vi "Periodic Tasks.vi"(8 "error in (no error)":errorcluster) -> ()   [LabVIEW 2019]
doc: "This VI runs in parallel to other tasks. It can contain as many user-defined periodic loops as you need. These can carry out PID or other sorts of timed response."
uses:
  <vilib>/Rock Robotics/WPI/ThirdParty/Phoenix-LabVIEW/Motor Controller/Controls/CTRE_Phoenix_MotorControl_ControlMode.ctl
  <vilib>/Rock Robotics/WPI/Solenoid/WPI_SolenoidValue.ctl
  <vilib>/Rock Robotics/WPI/ThirdParty/Sensors/navX/_TypeDefs/FRIC_navX_DeviceNumbersTypeDef.ctl
  <vilib>/Rock Robotics/WPI/ThirdParty/Phoenix-LabVIEW/Motor Controller/Controls/CTRE_Phoenix_MotorControl_FeedbackDevice.ctl
  <vilib>/Rock Robotics/WPI/DriverStation/WPI_DriverStationRobotMode2.ctl
  Corsair_V1/Team Code/Climber Routine.ctl
  Corsair_V1/Team Code/Ball Routine.ctl
  TurretMode.ctl
  LabVIEW_is_Under_Control.lib/Util/Toggle/Change Detect.vi
  LabVIEW_is_Under_Control.lib/Util/Toggle/Change Detect Boolean.vi
  <vilib>/Rock Robotics/WPI/Utilities/WPI_GetSetVariantRefNum.vi
  MotorsGlobal.vi
  JoysticksGlobal.vi
  <vilib>/Rock Robotics/Network Tables/NT Read Number.vi
  <vilib>/Rock Robotics/WPI/Solenoid/WPI_SolenoidSetEnum.vi
  <vilib>/Rock Robotics/WPI/ThirdParty/Phoenix-LabVIEW/Motor Controller/Get/CTRE_Phoenix_MotorController_GetSelectedSensorData.vi
  Robot Global Data.vi
  <vilib>/Rock Robotics/Network Tables/NT Write Number.vi
  <vilib>/Rock Robotics/WPI/ThirdParty/Phoenix-LabVIEW/Motor Controller/Get/CTRE_Phoenix_MotorController_GetVoltage.vi
  Ball counter.ctl
panel:
  in  "Distancia de longshot":dbl
  in  "Corsair Control":T1(tab)
  in  "EnableFWPID":bool
  out "Voltage":dbl
  out "Voltage Output":cluster{"Percent Output":dbl}(graph)
  out "Velocity PIDF":T2(graph)
  in  "I Zone":dbl
  in  "D":dbl
  in  "I":dbl
  in  "P":dbl=1.0
  in  "kF":dbl=0.031
  in  "FWSetpoint":dbl
  out "Flywheel Encoder":i32
  out "LTAGainsON?":bool
  in  "Inner Goal Height":dbl=2.49
  in  "Camera Angle":dbl=20.0
  out "Distancia do Goal":dbl
  in  "Camera Height":dbl=0.5599999999999999
  out "Turret PID":cluster{"Setpoint":dbl, "Process variable":dbl}(graph)
  in  "TAGains":T3={"proportional gain (Kc)"=0.4, "integral time (Ti, min)"=0.0, "derivative time (Td, min)"=0.0} {"derivative time (Td, min)" format="%.3f"; "integral time (Ti, min)" format="%.3f"; "proportional gain (Kc)" format="%.3f"}
  in  "HTARange":cluster{"output high":dbl, "output low":dbl}={"output high"=0.5, "output low"=-0.5} {"output low" format="%.2f"; "output high" format="%.2f"}
  in  "MaxAngle":dbl=1000.0
  in  "TASetpoint":dbl
  in  "Minimum command":dbl=0.05
  out "Turret Out":dbl
  in  "TADisable Range":dbl
  in  "TAIntegral Range":dbl=10000.0
  in  "LTARange":cluster{"output high":dbl, "output low":dbl}={"output high"=0.35, "output low"=-0.35} {"output low" format="%.2f"; "output high" format="%.2f"}
  in  "MTARange":cluster{"output high":dbl, "output low":dbl}={"output high"=0.19999999999999996, "output low"=-0.19999999999999996} {"output low" format="%.2f"; "output high" format="%.2f"}
  in  "LTAGains":T3={"proportional gain (Kc)"=0.4, "integral time (Ti, min)"=0.0, "derivative time (Td, min)"=0.0} {"derivative time (Td, min)" format="%.3f"; "integral time (Ti, min)" format="%.3f"; "proportional gain (Kc)" format="%.3f"}
  in  "Setpoint Climber":dbl=-110.0
  in  "Reset Encoders":bool
  out "Current 4":dbl
  out "Motor Temperature 4":u8
  out "Current 3":dbl
  out "Motor Temperature 3":u8
  out "Current 2":dbl
  out "Motor Temperature 2":u8
  out "Current":dbl
  out "Motor Temperature":u8
  out "Left Encoder":dbl
  out "Right Encoder":dbl
  in  "Sensitivty":dbl=1.5
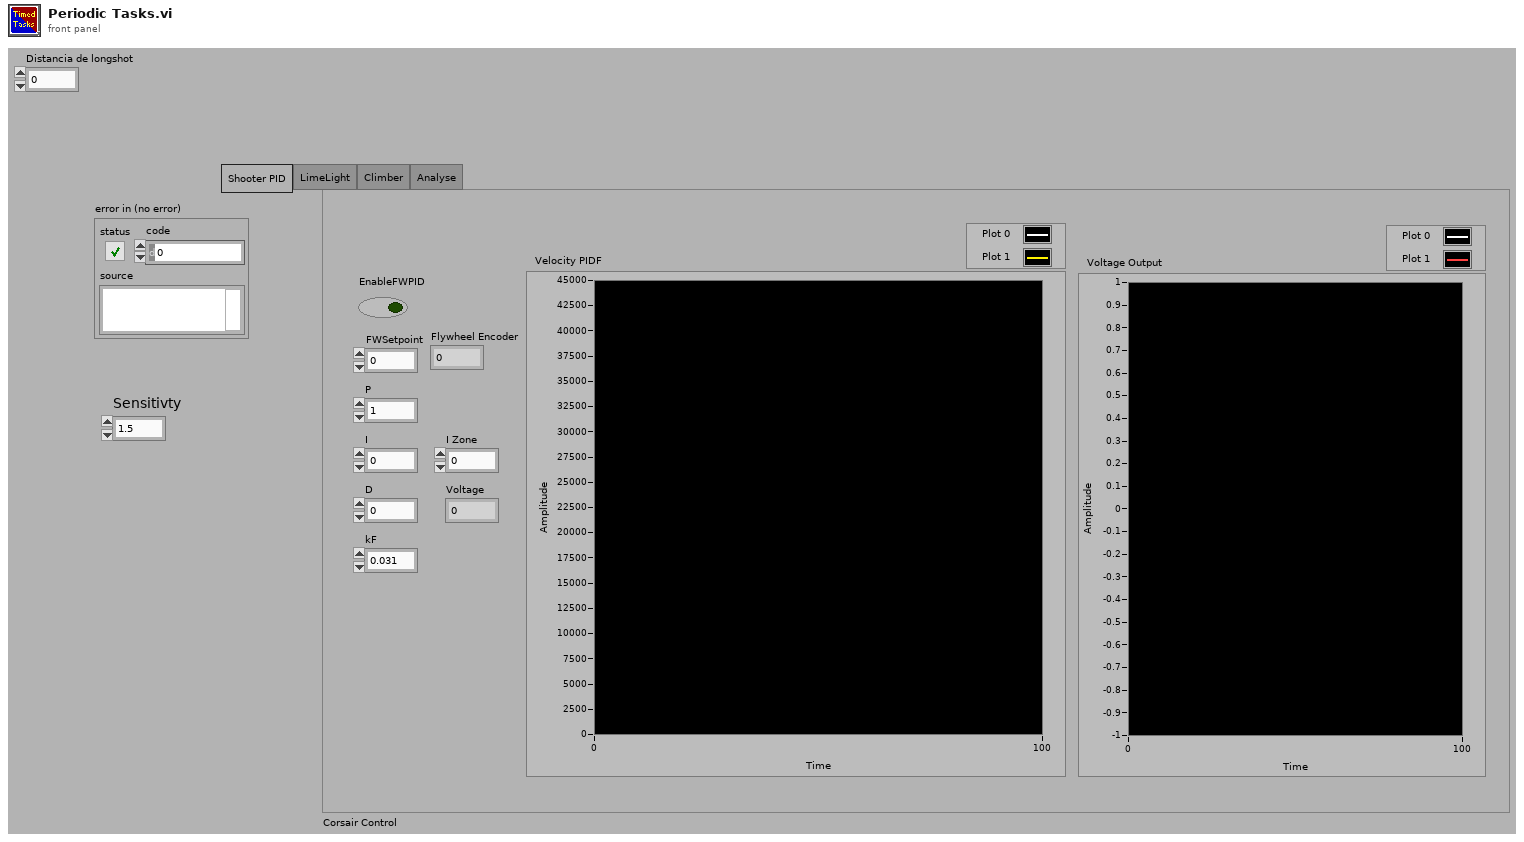
[diagram p1: front panel]
types:
  T1 = enum32{"Shooter PID", "LimeLight", "Climber", "Analyse"}
  T2 = cluster{"FWSetpoint":dbl, "Velocity (Raw Sensor Units per 100 ms)":i32}
  T3 = cluster{"proportional gain (Kc)":dbl, "integral time (Ti, min)":dbl, "derivative time (Td, min)":dbl}
  T4 = typedef "WPI_EncoderDevRef.ctl" = cluster{"DevStatus":errorcluster, "EncoderIndex":T5, "CounterIndex":T6, "DistancePerCount":dbl, "Decoding Type":T7}
  T5 = typedef "FPGA_EncoderIdx.ctl" = enum8{"Enc 0", "Enc 1", "Enc 2", "Enc 3", "Enc 4", "Enc 5", "Enc 6", "Enc 7", "Invalid"}
  T6 = typedef "FPGA_CounterCtrSystemIndex.ctl" = enum8{"Ctr 0", "Ctr 1", "Ctr 2", "Ctr 3", "Ctr 4", "Ctr 5", "Ctr 6", "Ctr 7", "Invalid"}
  T7 = typedef "WPI_EncoderType.ctl" = enum16{"1x", "2x", "4x"}
  T8 = typedef "WPI_JoystickDevRef.ctl" = cluster{"Device":T9}
  T9 = typedef "WPI_JoystickDeviceEnum.ctl" = enum16{"USB 0", "USB 1", "USB 2", "USB 3", "USB 4", "USB 5"}
  T10 = typedef "WPI_MotorControlDeviceRef.ctl" = cluster{"DeviceStatus":errorcluster, "Type":T11, "PWM":cluster{"PWM Channel":T12, "DeadBand":T13}, "CAN":cluster{"Device Number":u8, "SetOutput VI Ref":variant, "GetOutput VI Ref":variant, "Enable VI Ref":variant, "Disable VI Ref":variant, "Data":variant}, "Invert":bool, "DIO PWM":cluster{"PWM \"Enable\" Channel":T12, "DIOChannel":T14, "PWM Rate":dbl}}
  T11 = typedef "WPI_MotorControlType.ctl" = enum16{"PWM", "CAN", "DIO PWM"}
  T12 = typedef "FPGA_DIOPWMChannel.ctl" = enum8{"PWM 0", "PWM 1", "PWM 2", "PWM 3", "PWM 4", "PWM 5", "PWM 6", "PWM 7", "PWM 8", "PWM 9", "PWM MXP 0", "PWM MXP 1", "PWM MXP 2", "PWM MXP 3", "PWM MXP 4", "PWM MXP 5", "PWM MXP 6", "PWM MXP 7", "PWM MXP 8", "PWM MXP 9", "Invalid"}
  T13 = typedef "WPI_PWMDeadband.ctl" = cluster{"Name":string, "maxPositivePwm":i32, "minPositivePwm":i32, "centerPwm":i32, "maxNegativePwm":i32, "minNegativePwm":i32, "angularRange":u16}
  T14 = typedef "FPGA_DIOChannel.ctl" = enum8{"DIO 0", "DIO 1", "DIO 2", "DIO 3", "DIO 4", "DIO 5", "DIO 6", "DIO 7", "DIO 8", "DIO 9", "DIO MXP 0", "DIO MXP 1", "DIO MXP 2", "DIO MXP 3", "DIO MXP 4", "DIO MXP 5", "DIO MXP 6", "DIO MXP 7", "DIO MXP 8", "DIO MXP 9", "DIO MXP 10", "DIO MXP 11", "DIO MXP 12", "DIO MXP 13", "DIO MXP 14", "DIO MXP 15", "SPI Port CS1", "SPI Port CS2", "SPI Port CS3", "SPI Port MISO", "SPI Port MOSI", "Invalid"}
  T15 = typedef "WPI_SolenoidDevRef.ctl" = cluster{"DevStatus":errorcluster, "Pneumatics Control Module":u8, "Forward Solenoid Channel":T16, "Reverse Solenoid Channel":T16}
  T16 = typedef "WPI_SolenoidChannel.ctl" = enum8{"Solenoid 0", "Solenoid 1", "Solenoid 2", "Solenoid 3", "Solenoid 4", "Solenoid 5", "Solenoid 6", "Solenoid 7", "Invalid"}
  T17 = typedef "WPI_SwitchDevRef.ctl" = cluster{"DevStatus":errorcluster, "DIO Channel":T14, "CntIndex":T6, "Normally Closed":bool}
  T18 = typedef "FRIC_navX_DeviceNumbersTypeDef.ctl" = enum16{"Dev0", "Dev1", "Dev2", "Dev3"}
  T19 = typedef "WPI_SolenoidValue.ctl" = enum16{"Off", "On", "Forward", "Reverse"}
  T20 = typedef "CTRE_Phoenix_MotorControl_FeedbackDevice.ctl" = i8
  T21 = typedef "CTRE_Phoenix_MotorControl_ControlMode.ctl" = u16
  T22 = cluster{"Rollover":dbl, "Yaw":dbl, "Cont Yaw":dbl}
  T23 = typedef "WPI_DriverStationRobotMode2.ctl" = enum16{"Autonomous Disabled", "Autonomous Enabled", "Teleop Disabled", "Teleop Enabled", "Disconnected", "Finish", "Test Disabled", "Test Enabled", "Emergency Stopped"}
  T24 = typedef "WPI_RobotDriveDevRef.ctl" = cluster{"DevStatus":errorcluster, "Motors[]":T10[], "Square Inputs":bool, "Max Output":dbl}
  T25 = cluster{"Motors[][0]":T10, "Motors[][1]":T10, "Motors[][2]":T10, "Motors[][3]":T10, "Motors[][4]":T10, "Motors[][5]":T10, "Motors[][6]":T10, "Motors[][7]":T10, "Motors[][8]":T10}
  T26 = typedef "Ball Routine.ctl" = enum16{"Standart", "Get Power Cells", "Balls In", "Prepare Shooter", "Shoot!"}
  T27 = typedef "TurretMode.ctl" = enum16{"Static", "Manual", "Automatic"}
  T28 = typedef "Climber Routine.ctl" = enum16{"Standart", "Vibrate *Lenny Face*", "Open da Boi", "Engage on the Bar!", "Pull Our Hope", "Deu por Hoje"}
  T29 = typedef "Ball counter.ctl" = enum16{"Start", "More balls", "Less balls", "Ball! wait..."}
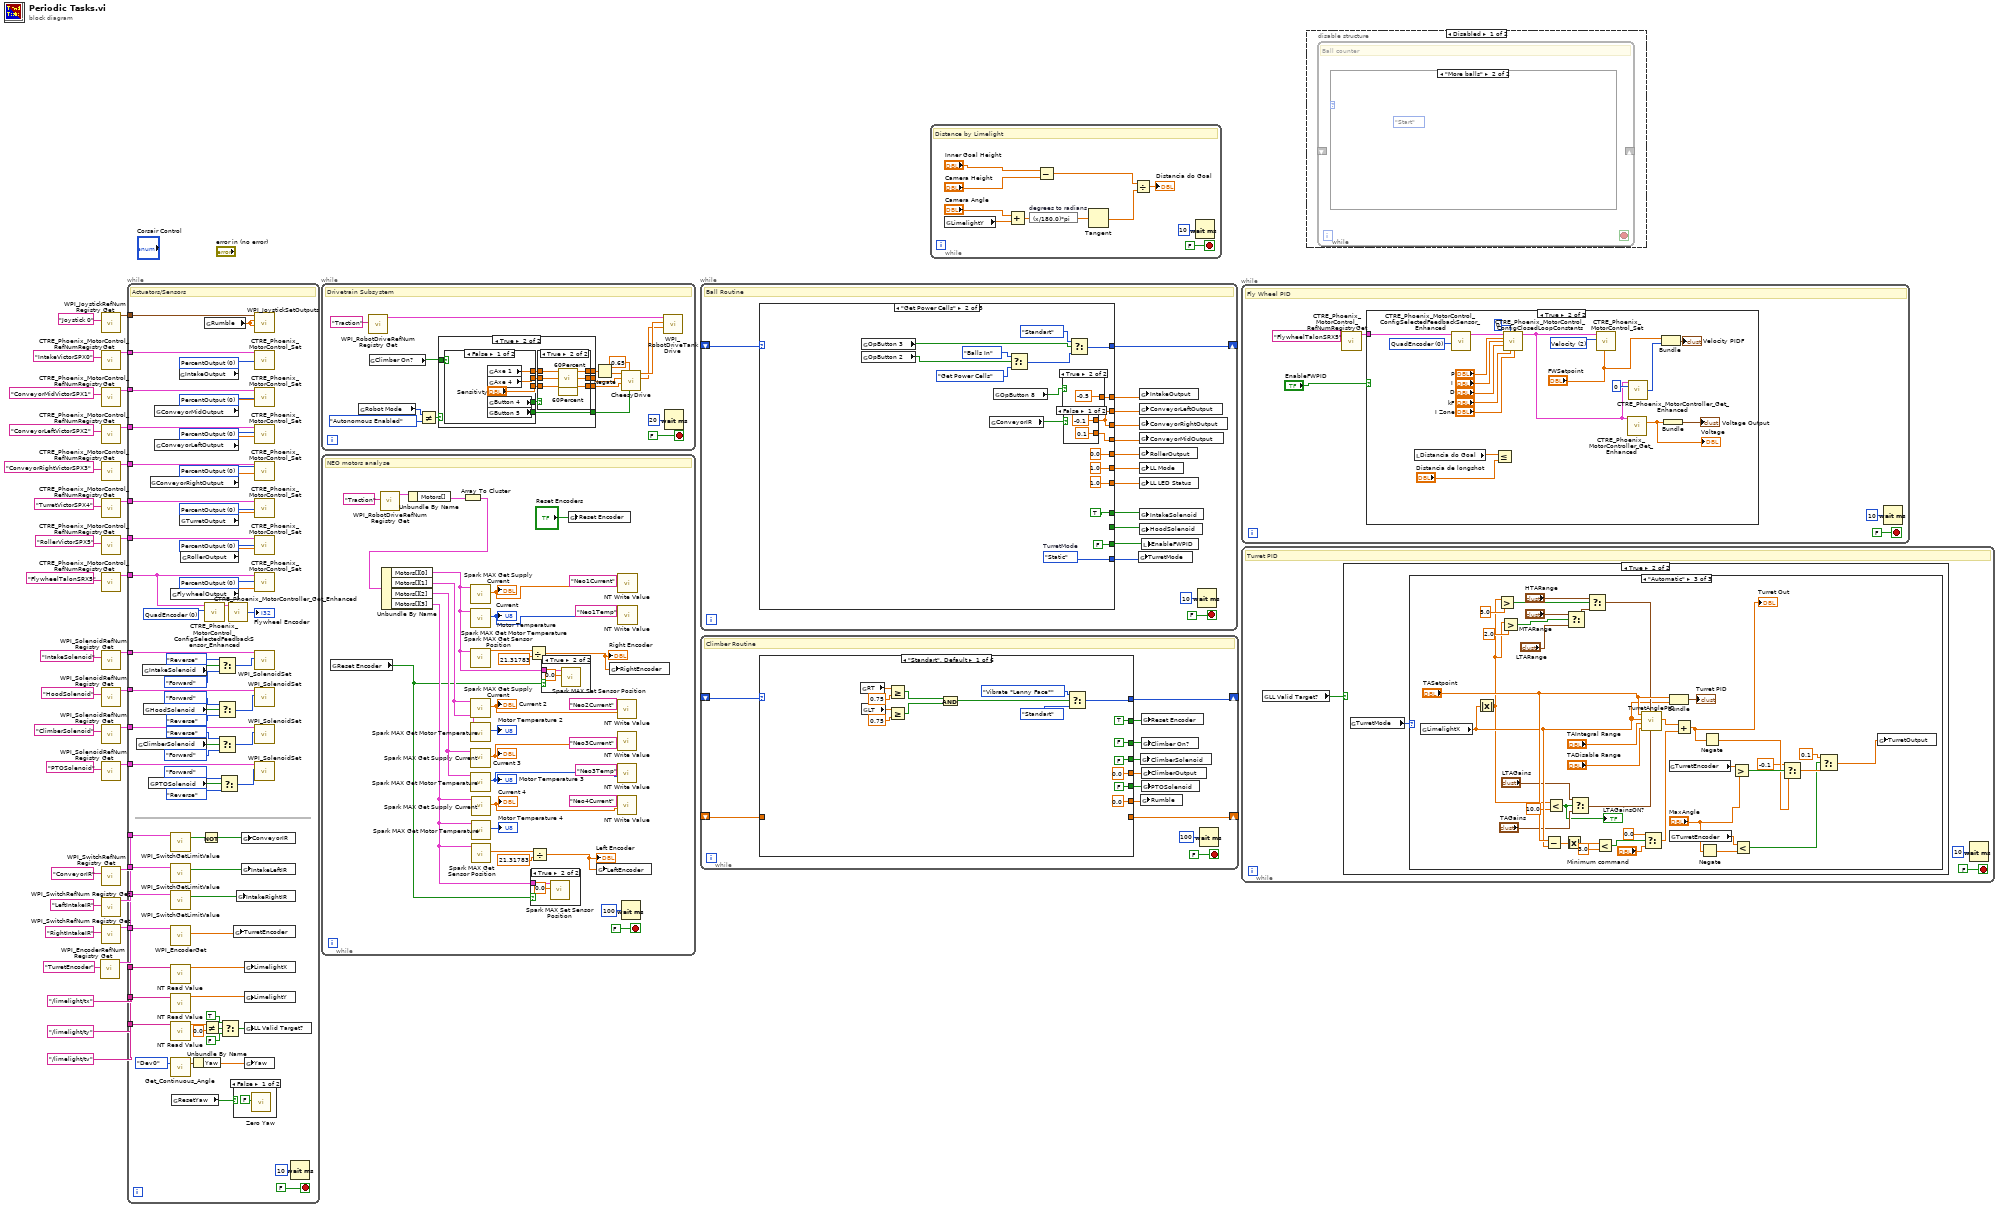
[diagram p0: block diagram]
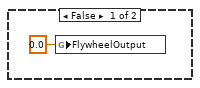
[diagram p4: hidden frame]
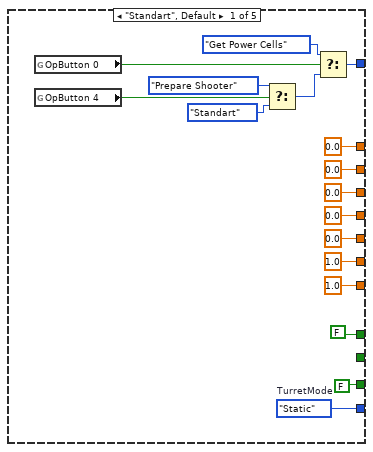
[diagram p5: hidden frame]
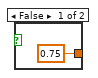
[diagram p6: hidden frame]
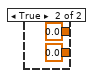
[diagram p7: hidden frame]
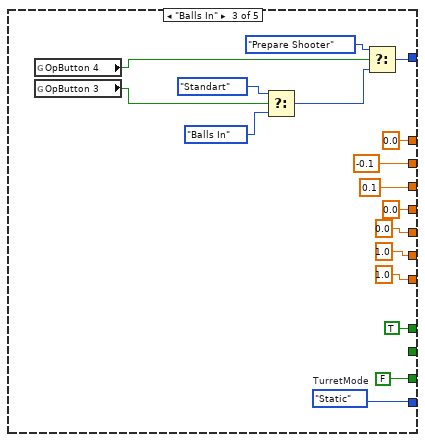
[diagram p8: hidden frame]
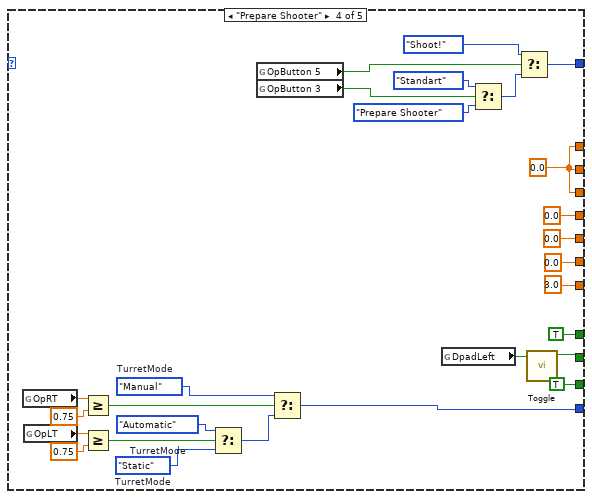
[diagram p9: hidden frame]
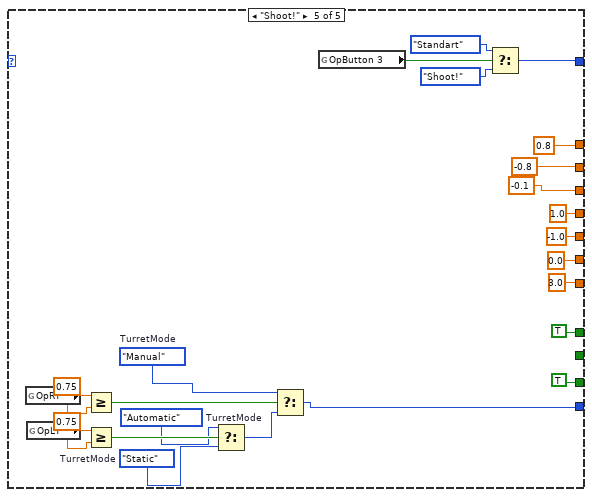
[diagram p10: hidden frame]
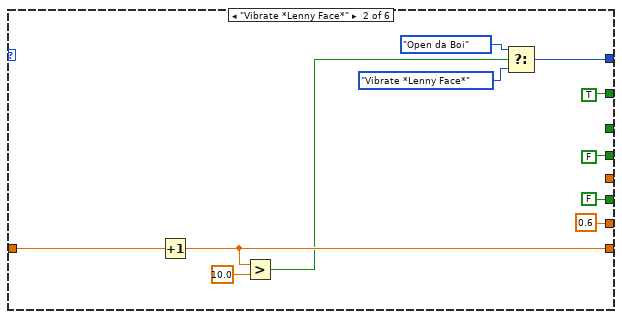
[diagram p11: hidden frame]
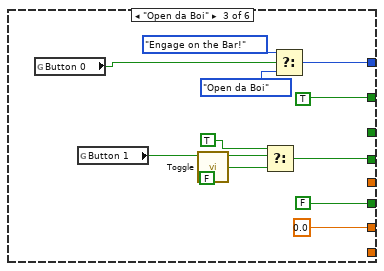
[diagram p12: hidden frame]
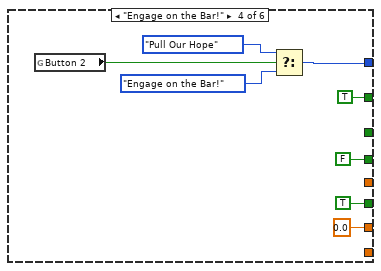
[diagram p13: hidden frame]
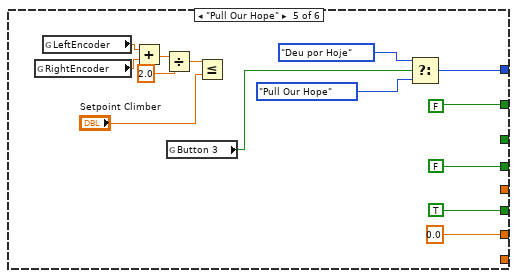
[diagram p14: hidden frame]
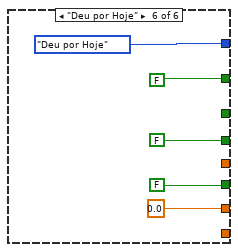
[diagram p15: hidden frame]
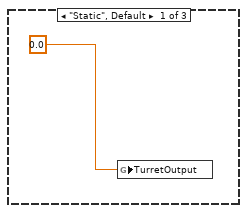
[diagram p17: hidden frame]
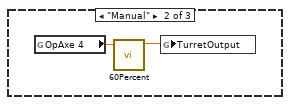
[diagram p18: hidden frame]
diagram:
  n1 = call <vilib>:"WPI_EncoderRefNum Registry Get.vi"("refnum name"="TurretEncoder") -> ("EncoderDevRef"=w5:T4)  [unwired: 9 in, 1 out]
  n2 = call <vilib>:"WPI_JoystickRefNum Registry Get.vi"("refnum name"="Joystick 0") -> ("JoystickDevRef"=w35:T8)  [unwired: 9 in, 1 out]
  n3 = call <vilib>:"CTRE_Phoenix_MotorControl_RefNumRegistryGet.vi"("refnum name"="IntakeVictorSPX0") -> ("PhoenixMotorControlDevRef"=w33:T10)  [unwired: 9 in, 1 out]
  n4 = call <vilib>:"CTRE_Phoenix_MotorControl_RefNumRegistryGet.vi"("refnum name"="ConveyorMidVictorSPX1") -> ("PhoenixMotorControlDevRef"=w30:T10)  [unwired: 9 in, 1 out]
  n5 = call <vilib>:"CTRE_Phoenix_MotorControl_RefNumRegistryGet.vi"("refnum name"="ConveyorLeftVictorSPX2") -> ("PhoenixMotorControlDevRef"=w29:T10)  [unwired: 9 in, 1 out]
  n6 = call <vilib>:"CTRE_Phoenix_MotorControl_RefNumRegistryGet.vi"("refnum name"="ConveyorRightVictorSPX3") -> ("PhoenixMotorControlDevRef"=w26:T10)  [unwired: 9 in, 1 out]
  n7 = call <vilib>:"CTRE_Phoenix_MotorControl_RefNumRegistryGet.vi"("refnum name"="TurretVictorSPX4") -> ("PhoenixMotorControlDevRef"=w25:T10)  [unwired: 9 in, 1 out]
  n8 = call <vilib>:"CTRE_Phoenix_MotorControl_RefNumRegistryGet.vi"("refnum name"="RollerVictorSPX5") -> ("PhoenixMotorControlDevRef"=w22:T10)  [unwired: 9 in, 1 out]
  n9 = call <vilib>:"CTRE_Phoenix_MotorControl_RefNumRegistryGet.vi"("refnum name"="FlywheelTalonSRX5") -> ("PhoenixMotorControlDevRef"=w21:T10)  [unwired: 9 in, 1 out]
  n10 = call <vilib>:"WPI_SolenoidRefNum Registry Get.vi"("refnum name"="IntakeSolenoid") -> ("SolenoidDevRef"=w19:T15)  [unwired: 9 in, 1 out]
  n11 = call <vilib>:"WPI_SolenoidRefNum Registry Get.vi"("refnum name"="HoodSolenoid") -> ("SolenoidDevRef"=w16:T15)  [unwired: 9 in, 1 out]
  n12 = call <vilib>:"WPI_SolenoidRefNum Registry Get.vi"("refnum name"="ClimberSolenoid") -> ("SolenoidDevRef"=w15:T15)  [unwired: 9 in, 1 out]
  n13 = call <vilib>:"WPI_SolenoidRefNum Registry Get.vi"("refnum name"="PTOSolenoid") -> ("SolenoidDevRef"=w12:T15)  [unwired: 9 in, 1 out]
  n14 = call <vilib>:"WPI_SwitchRefNum Registry Get.vi"("refnum name"="ConveyorIR") -> ("SwitchDevRef"=w7:T17)  [unwired: 9 in, 1 out]
  n15 = call <vilib>:"WPI_SwitchRefNum Registry Get.vi"("refnum name"="LeftIntakeIR") -> ("SwitchDevRef"=w4:T17)  [unwired: 9 in, 1 out]
  n16 = call <vilib>:"WPI_SwitchRefNum Registry Get.vi"("refnum name"="RightIntakeIR") -> ("SwitchDevRef"=w1:T17)  [unwired: 9 in, 1 out]
  n17 = while {
    tunnel: w35 -> [w105]
    tunnel: w33 -> [w103]
    tunnel: w30 -> [w99]
    tunnel: w29 -> [w98]
    tunnel: w26 -> [w93]
    tunnel: w25 -> [w92]
    tunnel: w22 -> [w87]
    tunnel: w21 -> [w45]
    tunnel: w19 -> [w83]
    tunnel: w16 -> [w76]
    tunnel: w15 -> [w73]
    tunnel: w12 -> [w66]
    tunnel: "/limelight/tx" ("Name") -> [w63]
    tunnel: "/limelight/tv" ("Name") -> [w55]
    tunnel: "/limelight/ty" ("Name") -> [w54]
    tunnel: w7 -> [w48]
    tunnel: w5 -> [w42]
    tunnel: w4 -> [w39]
    tunnel: w1 -> [w38]
    stop <- FALSE stop-if-true
    w43 = T20 0 items=["QuadEncoder"=0, "Analog"=2, "Tachometer"=4, "Pulse Width Encoded Position"=8, "Sensor Sum (S0 + S1)"=9, "Sensor Difference (D0 - D1)"=10, "Remote Source 0"=11, "Remote Source 1"=12, "Software Emulated"=15] ("Feedback Device")
    w86 = T21 0 items=["PercentOutput"=0, "Position"=1, "Velocity"=2, "Current"=3, "Follower"=5, "MotionProfile"=6, "MotionMagic"=7, "MotionProfileArc"=10, "Disabled"=15] ("Control Mode")
    w88 = T21 0 items=["PercentOutput"=0, "Position"=1, "Velocity"=2, "Current"=3, "Follower"=5, "MotionProfile"=6, "MotionMagic"=7, "MotionProfileArc"=10, "Disabled"=15] ("Control Mode")
    w91 = T21 0 items=["PercentOutput"=0, "Position"=1, "Velocity"=2, "Current"=3, "Follower"=5, "MotionProfile"=6, "MotionMagic"=7, "MotionProfileArc"=10, "Disabled"=15] ("Control Mode")
    w94 = T21 0 items=["PercentOutput"=0, "Position"=1, "Velocity"=2, "Current"=3, "Follower"=5, "MotionProfile"=6, "MotionMagic"=7, "MotionProfileArc"=10, "Disabled"=15] ("Control Mode")
    w97 = T21 0 items=["PercentOutput"=0, "Position"=1, "Velocity"=2, "Current"=3, "Follower"=5, "MotionProfile"=6, "MotionMagic"=7, "MotionProfileArc"=10, "Disabled"=15] ("Control Mode")
    w100 = T21 0 items=["PercentOutput"=0, "Position"=1, "Velocity"=2, "Current"=3, "Follower"=5, "MotionProfile"=6, "MotionMagic"=7, "MotionProfileArc"=10, "Disabled"=15] ("Control Mode")
    w102 = T21 0 items=["PercentOutput"=0, "Position"=1, "Velocity"=2, "Current"=3, "Follower"=5, "MotionProfile"=6, "MotionMagic"=7, "MotionProfileArc"=10, "Disabled"=15] ("Control Mode")
    # "Actuators/Sensors"
    n18 = global read "MotorsGlobal.vi" "ClimberSolenoid"() -> (w53:bool)
    n19 = global read "MotorsGlobal.vi" "IntakeSolenoid"() -> (w75:bool)
    n20 = global read "MotorsGlobal.vi" "HoodSolenoid"() -> (w74:bool)
    n21 = global read "MotorsGlobal.vi" "PTOSolenoid"() -> (w65:bool)
    n22 = global read "MotorsGlobal.vi" "ConveyorRightOutput"() -> (w95:dbl)
    n23 = global read "MotorsGlobal.vi" "ConveyorMidOutput"() -> (w101:dbl)
    n24 = global read "MotorsGlobal.vi" "ConveyorLeftOutput"() -> (w96:dbl)
    n25 = global read "MotorsGlobal.vi" "FlywheelOutput"() -> (w85:dbl)
    n26 = call <vilib>:"WPI_SwitchGetLimitValue.vi"("SwitchDevRef"=w48) -> ("Switch Pressed"=w47:bool)  [unwired: 8 in, 2 out]
    n27 = call <vilib>:"WPI_SwitchGetLimitValue.vi"("SwitchDevRef"=w39) -> ("Switch Pressed"=w40:bool)  [unwired: 8 in, 2 out]
    n28 = call <vilib>:"WPI_SwitchGetLimitValue.vi"("SwitchDevRef"=w38) -> ("Switch Pressed"=w37:bool)  [unwired: 8 in, 2 out]
    n29 = call <vilib>:"WPI_EncoderGet.vi"("EncoderDevRef"=w42) -> ("Distance"=w41:dbl)  [unwired: 5 in, 5 out]
    n30 = call-poly <vilib>:"NT Read Value.vi"("Name"=w63) -> ("Numeric"=w64:dbl)  [unwired: 9 in, 1 out]
    n31 = call-poly <vilib>:"NT Read Value.vi"("Name"=w54) -> ("Numeric"=w62:dbl)  [unwired: 9 in, 1 out]
    n32 = call-poly <vilib>:"NT Read Value.vi"("Name"=w55) -> ("Numeric"=w61:dbl)  [unwired: 9 in, 1 out]
    n33 = call <vilib>:"Get_Continuous_Angle.vi"("Device Number"=FRIC_navX_DeviceNumbersTypeDef."Dev0") -> ("Continuous Angle"=w52:T22)  [unwired: 10 in]
    n34 = global read "MotorsGlobal.vi" "ResetYaw"() -> (w49:bool)
    n35 = global read "MotorsGlobal.vi" "IntakeOutput"() -> (w84:dbl)
    n36 = global read "MotorsGlobal.vi" "TurretOutput"() -> (w90:dbl)
    n37 = global read "MotorsGlobal.vi" "RollerOutput"() -> (w89:dbl)
    n38 = Unbundle By Name(w52) -> ("Yaw"=w50:dbl)
    n39 = Not(x=w47) -> (.not. x?=w36:bool)
    n40 = Not Equal?(x=w61, y=0.0) -> (x != y?=w60:bool)
    n41 = global read "JoysticksGlobal.vi" "Rumble"() -> (w104:dbl)
    n42 = call <vilib>:"CTRE_Phoenix_MotorControl_ConfigSelectedFeedbackSensor_Enhanced.vi"("Feedback Device"=w43, "PhoenixMotorControlDevRef"=w45) -> ("PhoenixMotorControlDevRef"=w44:T10)  [unwired: 8 in, 1 out]
    n43 = Select(t=WPI_SolenoidValue."Reverse" ("Value"), s=w75, f=WPI_SolenoidValue."Forward" ("Value")) -> (s? t:f=w82:T19)
    n44 = Select(t=WPI_SolenoidValue."Forward" ("Value"), s=w74, f=WPI_SolenoidValue."Reverse" ("Value")) -> (s? t:f=w77:T19)
    n45 = Select(t=WPI_SolenoidValue."Reverse" ("Value"), s=w53, f=WPI_SolenoidValue."Forward" ("Value")) -> (s? t:f=w72:T19)
    n46 = Select(t=WPI_SolenoidValue."Forward" ("Value"), s=w65, f=WPI_SolenoidValue."Reverse" ("Value")) -> (s? t:f=w67:T19)
    n47 = Select(t=TRUE, s=w60, f=FALSE) -> (s? t:f=w59:bool)
    n48 = call-poly <vilib>:"CTRE_Phoenix_MotorController_Get_Enhanced.vi"("PhoenixMotorControlDevRef"=w44) -> ("Velocity (Raw Sensor Units per 100 ms)"=→"Flywheel Encoder":i32)  [unwired: 11 in, 3 out]
    n49 = case shown="False" w49 {
      frame False {
        n50 = call <vilib>:"Zero Yaw.vi"("Zero"=FALSE) -> ()  [unwired: 11 in]
      }
      frame True {
        n51 = call <vilib>:"Zero Yaw.vi"("Zero"=TRUE) -> ()  [unwired: 11 in]
      }
    }
    n52 = global write "MotorsGlobal.vi" "TurretEncoder"(w41) -> ()
    n53 = global write "MotorsGlobal.vi" "IntakeRightIR"(w37) -> ()
    n54 = global write "MotorsGlobal.vi" "IntakeLeftIR"(w40) -> ()
    n55 = global write "MotorsGlobal.vi" "ConveyorIR"(w36) -> ()
    n56 = global write "MotorsGlobal.vi" "LimelightX"(w64) -> ()
    n57 = global write "MotorsGlobal.vi" "LimelightY"(w62) -> ()
    n58 = global write "MotorsGlobal.vi" "LL Valid Target?"(w59) -> ()
    n59 = global write "MotorsGlobal.vi" "Yaw"(w50) -> ()
    n60 = call <vilib>:"WPI_JoystickSetOutputs.vi"("Right Rumble"=w104, "Left Rumble"=w104, "JoystickDevRef"=w105) -> ()  [unwired: 7 in, 2 out]
    n61 = call <vilib>:"CTRE_Phoenix_MotorControl_Set.vi"("Output"=w84, "Control Mode"=w102, "PhoenixMotorControlDevRef"=w103) -> ()  [unwired: 7 in, 2 out]
    n62 = call <vilib>:"CTRE_Phoenix_MotorControl_Set.vi"("Output"=w101, "Control Mode"=w100, "PhoenixMotorControlDevRef"=w99) -> ()  [unwired: 7 in, 2 out]
    n63 = call <vilib>:"CTRE_Phoenix_MotorControl_Set.vi"("Output"=w96, "Control Mode"=w97, "PhoenixMotorControlDevRef"=w98) -> ()  [unwired: 7 in, 2 out]
    n64 = call <vilib>:"CTRE_Phoenix_MotorControl_Set.vi"("Output"=w95, "Control Mode"=w94, "PhoenixMotorControlDevRef"=w93) -> ()  [unwired: 7 in, 2 out]
    n65 = call <vilib>:"CTRE_Phoenix_MotorControl_Set.vi"("Output"=w90, "Control Mode"=w91, "PhoenixMotorControlDevRef"=w92) -> ()  [unwired: 7 in, 2 out]
    n66 = call <vilib>:"CTRE_Phoenix_MotorControl_Set.vi"("Output"=w89, "Control Mode"=w88, "PhoenixMotorControlDevRef"=w87) -> ()  [unwired: 7 in, 2 out]
    n67 = call <vilib>:"CTRE_Phoenix_MotorControl_Set.vi"("Output"=w85, "Control Mode"=w86, "PhoenixMotorControlDevRef"=w45) -> ()  [unwired: 7 in, 2 out]
    n68 = call-poly <vilib>:"WPI_SolenoidSet.vi"("Value"=w82, "SolenoidDevRef"=w83) -> ()  [unwired: 8 in, 2 out]
    n69 = call-poly <vilib>:"WPI_SolenoidSet.vi"("Value"=w77, "SolenoidDevRef"=w76) -> ()  [unwired: 8 in, 2 out]
    n70 = call-poly <vilib>:"WPI_SolenoidSet.vi"("Value"=w72, "SolenoidDevRef"=w73) -> ()  [unwired: 8 in, 2 out]
    n71 = call-poly <vilib>:"WPI_SolenoidSet.vi"("Value"=w67, "SolenoidDevRef"=w66) -> ()  [unwired: 8 in, 2 out]
    n72 = Wait (ms)(milliseconds to wait=u32 10) -> ()  [unwired: 1 out]
  }
  n73 = while {
    stop <- FALSE stop-if-true
    # "Drivetrain Subsystem"
    n74 = global read "Robot Global Data.vi" "Robot Mode"() -> (w110:T23)
    n75 = call <vilib>:"WPI_RobotDriveRefNum Registry Get.vi"("refnum name"="Traction") -> ("RobotDriveDevRef"=w123:T24)  [unwired: 9 in, 1 out]
    n76 = global read "MotorsGlobal.vi" "Climber On?"() -> (w113:bool)
    n77 = Not Equal?(x=w110, y=WPI_DriverStationRobotMode2."Autonomous Enabled" ("Robot Mode")) -> (x != y?=w112:bool)
    n78 = case shown="True" w112 {
      tunnel: [w128 w138] -> w121
      tunnel: [TRUE ("Button 5") w133] -> w120
      tunnel: [1.0 ("Sensitivty") w132] -> w118
      tunnel: [w129 w131] -> w117
      tunnel: w113 -> [_ w130]
      frame False {
        n79 = global read "JoysticksGlobal.vi" "AutoAxe1"() -> (w128:dbl)
        n80 = global read "JoysticksGlobal.vi" "AutoAxe4"() -> (w129:dbl)
      }
      frame True {
        n81 = case shown="False" w130 {
          tunnel: [w143 w148] -> w137
          tunnel: [w142 0.0 ("Axe 4")] -> w136
          tunnel: [w141 FALSE ("Button 4")] -> w135
          tunnel: ["Sensitivty" 1.0 ("Sensitivty")] -> w134
          tunnel: [w139 FALSE ("Button 5")] -> w133
          frame False {
            n82 = global read "JoysticksGlobal.vi" "Axe 1"() -> (w143:dbl)
            n83 = global read "JoysticksGlobal.vi" "Axe 4"() -> (w142:dbl)
            n84 = global read "JoysticksGlobal.vi" "Button 4"() -> (w141:bool)
            n85 = global read "JoysticksGlobal.vi" "Button 5"() -> (w139:bool)
          }
          frame True {
            n86 = global read "MotorsGlobal.vi" "ClimberOutput"() -> (w148:dbl)
          }
        }
        n87 = case shown="True" w135 {
          tunnel: [w151 w156] -> w138
          tunnel: [w150 w155] -> w131
          tunnel: w137 -> [w151 w154]
          tunnel: w136 -> [w150 w153]
          tunnel: [w149 w152] -> w132
          tunnel: w134 -> [w149 w152]
          frame False {
          }
          frame True {
            n88 = call "60Percent.vi"("In"=w154) -> ("Out"=w156:dbl)  [unwired: 9 in]
            n89 = call "60Percent.vi"("In"=w153) -> ("Out"=w155:dbl)  [unwired: 9 in]
          }
        }
      }
    }
    n90 = Negate(x=w121) -> (-x=w116:dbl)
    n91 = call "CheesyDrive.vi"("Quickturn"=w120, "WheelNonLinearity"=0.65, "Sensitivty"=w118, "Wheel"=w117, "Throttle"=w116) -> ("Right PWM"=w114:dbl, "Left PWM"=w115:dbl)  [unwired: 5 in]
    n92 = call <vilib>:"WPI_RobotDriveTankDrive.vi"("Right axis value"=w114, "Left axis value"=w115, "RobotDriveDevRef"=w123) -> ()  [unwired: 6 in, 3 out]
    n93 = Wait (ms)(milliseconds to wait=u32 20) -> ()  [unwired: 1 out]
  }
  n94 = while {
    stop <- FALSE stop-if-true
    # "NEO motors analyse"
    n95 = global read "MotorsGlobal.vi" "Reset Encoder"() -> (w164:bool)
    n96 = call <vilib>:"WPI_RobotDriveRefNum Registry Get.vi"("refnum name"="Traction") -> ("RobotDriveDevRef"=w187:T24)  [unwired: 9 in, 1 out]
    n97 = Unbundle By Name(w187) -> ("Motors[]"=w186:T10[])
    n98 = Array To Cluster(array=w186) -> (cluster=w181:T25)
    n99 = Unbundle By Name(w181) -> ("Motors[][0]"=w166:T10, "Motors[][1]"=w180:T10, "Motors[][2]"=w179:T10, "Motors[][3]"=w165:T10)
    n100 = call <vilib>:"Spark MAX Get Supply Current.vi"("MotorControlDevRef in"=w166) -> ("Current"=w177:dbl)  [unwired: 7 in, 3 out]
    "Current" <- w177
    n101 = call <vilib>:"Spark MAX Get Motor Temperature.vi"("MotorControlDevRef in"=w166) -> ("Motor Temperature"=w175:u8)  [unwired: 7 in, 3 out]
    "Motor Temperature" <- w175
    n102 = call <vilib>:"Spark MAX Get Sensor Position.vi"("MotorControlDevRef in"=w166) -> ("Sensor Position"=w161:dbl)  [unwired: 7 in, 3 out]
    n103 = call <vilib>:"Spark MAX Get Supply Current.vi"("MotorControlDevRef in"=w180) -> ("Current"=w174:dbl)  [unwired: 7 in, 3 out]
    "Current 2" <- w174
    n104 = call <vilib>:"Spark MAX Get Motor Temperature.vi"("MotorControlDevRef in"=w180) -> ("Motor Temperature"=→"Motor Temperature 2":u8)  [unwired: 7 in, 3 out]
    n105 = call <vilib>:"Spark MAX Get Supply Current.vi"("MotorControlDevRef in"=w179) -> ("Current"=w173:dbl)  [unwired: 7 in, 3 out]
    "Current 3" <- w173
    n106 = call <vilib>:"Spark MAX Get Motor Temperature.vi"("MotorControlDevRef in"=w179) -> ("Motor Temperature"=w172:u8)  [unwired: 7 in, 3 out]
    "Motor Temperature 3" <- w172
    n107 = call <vilib>:"Spark MAX Get Supply Current.vi"("MotorControlDevRef in"=w165) -> ("Current"=w171:dbl)  [unwired: 7 in, 3 out]
    "Current 4" <- w171
    n108 = call <vilib>:"Spark MAX Get Motor Temperature.vi"("MotorControlDevRef in"=w165) -> ("Motor Temperature"=→"Motor Temperature 4":u8)  [unwired: 7 in, 3 out]
    n109 = call <vilib>:"Spark MAX Get Sensor Position.vi"("MotorControlDevRef in"=w165) -> ("Sensor Position"=w159:dbl)  [unwired: 7 in, 3 out]
    n110 = Divide(x=w161, y=21.31783) -> (x/y=w160:dbl)
    "Right Encoder" <- w160
    n111 = Divide(x=w159, y=21.31783) -> (x/y=w157:dbl)
    "Left Encoder" <- w157
    n112 = case shown="True" w164 {
      tunnel: w165 -> [_ w190]
      frame False {
      }
      frame True {
        n113 = call <vilib>:"Spark MAX Set Sensor Position.vi"("Position"=0.0, "MotorControlDeviceRef"=w190) -> ()  [unwired: 8 in, 2 out]
      }
    }
    n114 = case shown="True" w164 {
      tunnel: w166 -> [_ w192]
      frame False {
      }
      frame True {
        n115 = call <vilib>:"Spark MAX Set Sensor Position.vi"("Position"=0.0, "MotorControlDeviceRef"=w192) -> ()  [unwired: 8 in, 2 out]
      }
    }
    n116 = global write "MotorsGlobal.vi" "Reset Encoder"("Reset Encoders") -> ()
    n117 = global write "MotorsGlobal.vi" "LeftEncoder"(w157) -> ()
    n118 = global write "MotorsGlobal.vi" "RightEncoder"(w160) -> ()
    n119 = call-poly <vilib>:"NT Write Value.vi"("Numeric"=w174, "Name"="Neo2Current") -> ()  [unwired: 9 in, 1 out]
    n120 = call-poly <vilib>:"NT Write Value.vi"("Numeric"=w173, "Name"="Neo3Current") -> ()  [unwired: 9 in, 1 out]
    n121 = call-poly <vilib>:"NT Write Value.vi"("Numeric"=w172, "Name"="Neo3Temp") -> ()  [unwired: 9 in, 1 out]
    n122 = call-poly <vilib>:"NT Write Value.vi"("Numeric"=w171, "Name"="Neo4Current") -> ()  [unwired: 9 in, 1 out]
    n123 = call-poly <vilib>:"NT Write Value.vi"("Numeric"=w177, "Name"="Neo1Current") -> ()  [unwired: 9 in, 1 out]
    n124 = call-poly <vilib>:"NT Write Value.vi"("Numeric"=w175, "Name"="Neo1Temp") -> ()  [unwired: 9 in, 1 out]
    n125 = Wait (ms)(milliseconds to wait=u32 100) -> ()  [unwired: 1 out]
  }
  n126 = while {
    shift-right: [w204] -> _
    shift-left: _ -> [w205]
    stop <- FALSE stop-if-true
    # "Ball Routine"
    n127 = case shown="\"Get Power Cells\"" w205 {
      tunnel: [w224 w240 w264 w289 w312] -> w204
      tunnel: [0.0 w241 0.0 w266 0.8] -> w203
      tunnel: [0.0 0.0 0.0 0.0 -1.0] -> w202
      tunnel: [0.0 w235 -0.1 w266 -0.8] -> w201
      tunnel: [0.0 w235 0.1 w266 -0.1] -> w200
      tunnel: [0.0 w234 0.0 0.0 1.0] -> w199
      tunnel: [FALSE ("IntakeSolenoid") TRUE ("IntakeSolenoid") TRUE ("IntakeSolenoid") TRUE ("IntakeSolenoid") TRUE ("IntakeSolenoid")] -> w194
      tunnel: [_ _ _ w291 _] -> w198
      tunnel: [1.0 1.0 1.0 3.0 3.0] -> w197
      tunnel: [1.0 1.0 1.0 0.0 0.0] -> w196
      tunnel: [FALSE ("IntakeSolenoid") FALSE ("IntakeSolenoid") FALSE ("IntakeSolenoid") TRUE ("IntakeSolenoid") TRUE ("IntakeSolenoid")] -> w195
      tunnel: [w208 w232 w250 w267 w296] -> w193
      frame "Standart", Default {
        w208 = TurretMode."Static"  # TurretMode
        n128 = global read "JoysticksGlobal.vi" "OpButton 0"() -> (w212:bool)
        n129 = global read "JoysticksGlobal.vi" "OpButton 4"() -> (w213:bool)
        n130 = Select(t=Ball_Routine."Prepare Shooter", s=w213, f=Ball_Routine."Standart") -> (s? t:f=w216:T26)
        n131 = Select(t=Ball_Routine."Get Power Cells", s=w212, f=w216) -> (s? t:f=w224:T26)
      }
      frame "Get Power Cells" {
        w232 = TurretMode."Static"  # TurretMode
        n132 = global read "JoysticksGlobal.vi" "OpButton 3"() -> (w228:bool)
        n133 = global read "JoysticksGlobal.vi" "OpButton 2"() -> (w227:bool)
        n134 = global read "MotorsGlobal.vi" "ConveyorIR"() -> (w225:bool)
        n135 = global read "JoysticksGlobal.vi" "OpButton 8"() -> (w226:bool)
        n136 = Select(t=Ball_Routine."Balls In", s=w227, f=Ball_Routine."Get Power Cells") -> (s? t:f=w230:T26)
        n137 = case shown="True" w226 {
          tunnel: [0.75 -0.5] -> w241
          frame False {
          }
          frame True {
          }
        }
        n138 = case shown="False" w225 {
          tunnel: [-0.1 0.0] -> w235
          tunnel: [0.1 0.0] -> w234
          frame False {
          }
          frame True {
          }
        }
        n139 = Select(t=Ball_Routine."Standart", s=w228, f=w230) -> (s? t:f=w240:T26)
      }
      frame "Balls In" {
        w250 = TurretMode."Static"  # TurretMode
        n140 = global read "JoysticksGlobal.vi" "OpButton 4"() -> (w259:bool)
        n141 = global read "JoysticksGlobal.vi" "OpButton 3"() -> (w260:bool)
        n142 = Select(t=Ball_Routine."Standart", s=w260, f=Ball_Routine."Balls In") -> (s? t:f=w263:T26)
        n143 = Select(t=Ball_Routine."Prepare Shooter", s=w259, f=w263) -> (s? t:f=w264:T26)
      }
      frame "Prepare Shooter" {
        w272 = TurretMode."Manual"  # TurretMode
        w270 = TurretMode."Automatic"  # TurretMode
        w271 = TurretMode."Static"  # TurretMode
        w266 = 0.0
        n144 = global read "JoysticksGlobal.vi" "OpRT"() -> (w275:dbl)
        n145 = global read "JoysticksGlobal.vi" "OpLT"() -> (w274:dbl)
        n146 = Greater Or Equal?(x=w275, y=0.75) -> (x >= y?=w277:bool)
        n147 = Greater Or Equal?(x=w274, y=0.75) -> (x >= y?=w276:bool)
        n148 = Select(t=w270, s=w276, f=w271) -> (s? t:f=w273:T27)
        n149 = global read "JoysticksGlobal.vi" "OpButton 5"() -> (w288:bool)
        n150 = global read "JoysticksGlobal.vi" "OpButton 3"() -> (w286:bool)
        n151 = Select(t=w272, s=w277, f=w273) -> (s? t:f=w267:T27)
        n152 = global read "JoysticksGlobal.vi" "DpadLeft"() -> (w292:bool)
        n153 = Select(t=Ball_Routine."Standart", s=w286, f=Ball_Routine."Prepare Shooter") -> (s? t:f=w287:T26)
        n154 = Select(t=Ball_Routine."Shoot!", s=w288, f=w287) -> (s? t:f=w289:T26)
        n155 = call "Toggle.vi"("In"=w292) -> ("Toggled"=w291:bool)  [unwired: 10 in]
      }
      frame "Shoot!" {
        w301 = TurretMode."Manual"  # TurretMode
        w299 = TurretMode."Automatic"  # TurretMode
        w300 = TurretMode."Static"  # TurretMode
        n156 = global read "JoysticksGlobal.vi" "OpRT"() -> (w304:dbl)
        n157 = global read "JoysticksGlobal.vi" "OpLT"() -> (w303:dbl)
        n158 = Greater Or Equal?(x=w304, y=0.75) -> (x >= y?=w306:bool)
        n159 = Greater Or Equal?(x=w303, y=0.75) -> (x >= y?=w305:bool)
        n160 = Select(t=w299, s=w305, f=w300) -> (s? t:f=w302:T27)
        n161 = Select(t=w301, s=w306, f=w302) -> (s? t:f=w296:T27)
        n162 = global read "JoysticksGlobal.vi" "OpButton 3"() -> (w314:bool)
        n163 = Select(t=Ball_Routine."Standart", s=w314, f=Ball_Routine."Shoot!") -> (s? t:f=w312:T26)
      }
    }
    n164 = global write "MotorsGlobal.vi" "TurretMode"(w193) -> ()
    n165 = global write "MotorsGlobal.vi" "IntakeOutput"(w203) -> ()
    n166 = global write "MotorsGlobal.vi" "ConveyorLeftOutput"(w201) -> ()
    n167 = global write "MotorsGlobal.vi" "ConveyorRightOutput"(w200) -> ()
    n168 = global write "MotorsGlobal.vi" "ConveyorMidOutput"(w199) -> ()
    n169 = global write "MotorsGlobal.vi" "RollerOutput"(w202) -> ()
    n170 = global write "MotorsGlobal.vi" "LL Mode"(w196) -> ()
    n171 = global write "MotorsGlobal.vi" "LL LED Status"(w197) -> ()
    n172 = global write "MotorsGlobal.vi" "IntakeSolenoid"(w194) -> ()
    n173 = global write "MotorsGlobal.vi" "HoodSolenoid"(w198) -> ()
    n174 = local write "EnableFWPID"(w195) -> ()
    n175 = Wait (ms)(milliseconds to wait=u32 10) -> ()  [unwired: 1 out]
  }
  n176 = while {
    shift-right: [w325] -> _
    shift-left: _ -> [w324]
    shift-right: [w321] -> _
    shift-left: _ -> [w322]
    stop <- FALSE stop-if-true
    # "Climber Routine"
    n177 = case shown="\"Standart\", Default" w324 {
      tunnel: [FALSE FALSE w361 FALSE FALSE FALSE] -> w326
      tunnel: [w341 w354 w366 w370 w381 Climber_Routine."Deu por Hoje"] -> w325
      tunnel: [0.0 0.6 0.0 0.0 0.0 0.0] -> w323
      tunnel: w322 -> [_ w353 _ _ _ _]
      tunnel: [_ w352 _ _ _ _] -> w321
      tunnel: [FALSE FALSE FALSE TRUE TRUE FALSE] -> w320
      tunnel: [TRUE ("Reset Encoder") TRUE ("Reset Encoder") TRUE ("Reset Encoder") TRUE ("Reset Encoder") FALSE ("Reset Encoder") FALSE ("Reset Encoder")] -> w319
      tunnel: [0.0 ("ClimberOutput") _ _ _ _ _] -> w318
      tunnel: [FALSE ("Climber On?") _ _ _ _ _] -> w317
      frame "Standart", Default {
        n178 = global read "JoysticksGlobal.vi" "RT"() -> (w337:dbl)
        n179 = global read "JoysticksGlobal.vi" "LT"() -> (w336:dbl)
        n180 = Greater Or Equal?(x=w337, y=0.75) -> (x >= y?=w333:bool)
        n181 = Greater Or Equal?(x=w336, y=0.75) -> (x >= y?=w332:bool)
        n182 = And(x=w333, y=w332) -> (x .and. y?=w343:bool)
        n183 = Select(t=Climber_Routine."Vibrate *Lenny Face*", s=w343, f=Climber_Routine."Standart") -> (s? t:f=w341:T28)
      }
      frame "Vibrate *Lenny Face*" {
        n184 = Increment(x=w353) -> (x+1=w352:dbl)
        n185 = Greater?(x=w352, y=10.0) -> (0:w350:bool)
        n186 = Select(t=Climber_Routine."Open da Boi", s=w350, f=Climber_Routine."Vibrate *Lenny Face*") -> (s? t:f=w354:T28)
      }
      frame "Open da Boi" {
        n187 = global read "JoysticksGlobal.vi" "Button 0"() -> (w363:bool)
        n188 = global read "JoysticksGlobal.vi" "Button 1"() -> (w357:bool)
        n189 = call "Toggle.vi"("In"=w357) -> ("Toggled"=w358:bool)  [unwired: 10 in]
        n190 = Select(t=TRUE, s=w358, f=FALSE) -> (s? t:f=w361:bool)
        n191 = Select(t=Climber_Routine."Engage on the Bar!", s=w363, f=Climber_Routine."Open da Boi") -> (s? t:f=w366:T28)
      }
      frame "Engage on the Bar!" {
        n192 = global read "JoysticksGlobal.vi" "Button 2"() -> (w371:bool)
        n193 = Select(t=Climber_Routine."Pull Our Hope", s=w371, f=Climber_Routine."Engage on the Bar!") -> (s? t:f=w370:T28)
      }
      frame "Pull Our Hope" {
        n194 = global read "MotorsGlobal.vi" "RightEncoder"() -> (w379:dbl)
        n195 = global read "MotorsGlobal.vi" "LeftEncoder"() -> (w378:dbl)
        n196 = Add(x=w378, y=w379) -> (x+y=w387:dbl)
        n197 = Divide(x=w387, y=2.0) -> (x/y=w385:dbl)
        n198 = global read "JoysticksGlobal.vi" "Button 3"() -> (w376:bool)
        n199 = Less Or Equal?(x=w385, y="Setpoint Climber") -> ()  [unwired: 1 out]
        n200 = Select(t=Climber_Routine."Deu por Hoje", s=w376, f=Climber_Routine."Pull Our Hope") -> (s? t:f=w381:T28)
      }
      frame "Deu por Hoje" {
      }
    }
    n201 = global write "MotorsGlobal.vi" "ClimberSolenoid"(w326) -> ()
    n202 = global write "JoysticksGlobal.vi" "Rumble"(w323) -> ()
    n203 = global write "MotorsGlobal.vi" "Reset Encoder"(w319) -> ()
    n204 = global write "MotorsGlobal.vi" "Climber On?"(w317) -> ()
    n205 = global write "MotorsGlobal.vi" "ClimberOutput"(w318) -> ()
    n206 = global write "MotorsGlobal.vi" "PTOSolenoid"(w320) -> ()
    n207 = Wait (ms)(milliseconds to wait=u32 100) -> ()  [unwired: 1 out]
  }
  n208 = while {
    stop <- FALSE stop-if-true
    # "Distance by Limelight"
    n209 = global read "MotorsGlobal.vi" "LimelightY"() -> (w395:dbl)
    n210 = Add(x="Camera Angle", y=w395) -> (x+y=w397:dbl)
    n211 = expression code="(x/180.0)*pi" "degrees to radians"(w397) -> (w398:dbl)
    n212 = Subtract(x="Inner Goal Height", y="Camera Height") -> (x-y=w404:dbl)
    n213 = Tangent(1:w398) -> (0:w405:dbl)
    n214 = Divide(x=w404, y=w405) -> (x/y=→"Distancia do Goal":dbl)
    n215 = Wait (ms)(milliseconds to wait=u32 10) -> ()  [unwired: 1 out]
  }
  n216 = while {
    stop <- FALSE stop-if-true
    # "Fly Wheel PID"
    n217 = call <vilib>:"CTRE_Phoenix_MotorControl_RefNumRegistryGet.vi"("refnum name"="FlywheelTalonSRX5") -> ("PhoenixMotorControlDevRef"=w407:T10)  [unwired: 9 in, 1 out]
    n218 = case shown="True" "EnableFWPID" {
      tunnel: w407 -> [_ w430]
      frame False {
        n219 = global write "MotorsGlobal.vi" "FlywheelOutput"(0.0 ("FlywheelOutput")) -> ()
      }
      frame True {
        w421 = T21 2 items=["PercentOutput"=0, "Position"=1, "Velocity"=2, "Current"=3, "Follower"=5, "MotionProfile"=6, "MotionMagic"=7, "MotionProfileArc"=10, "Disabled"=15] ("Control Mode")
        w429 = T20 0 items=["QuadEncoder"=0, "Analog"=2, "Tachometer"=4, "Pulse Width Encoded Position"=8, "Sensor Sum (S0 + S1)"=9, "Sensor Difference (D0 - D1)"=10, "Remote Source 0"=11, "Remote Source 1"=12, "Software Emulated"=15] ("Feedback Device")
        n220 = local read "Distancia do Goal"() -> (w415:dbl)
        n221 = call <vilib>:"CTRE_Phoenix_MotorControl_ConfigSelectedFeedbackSensor_Enhanced.vi"("Feedback Device"=w429, "PhoenixMotorControlDevRef"=w430) -> ("PhoenixMotorControlDevRef"=w428:T10)  [unwired: 8 in, 1 out]
        n222 = Less Or Equal?(x=w415, y="Distancia de longshot") -> ()  [unwired: 1 out]
        n223 = call <vilib>:"CTRE_Phoenix_MotorControl_ConfigClosedLoopConstants.vi"("PhoenixMotorControlDevRef"=w428, "slotIdx"=0, "P"="P", "I"="I", "D"="D", "F"="kF", "I Zone"="I Zone") -> ("PhoenixMotorControlDevRef"=w413:T10)  [unwired: 7 in, 1 out]
        n224 = call <vilib>:"CTRE_Phoenix_MotorControl_Set.vi"("Output"="FWSetpoint", "Control Mode"=w421, "PhoenixMotorControlDevRef"=w413) -> ()  [unwired: 7 in, 2 out]
        n225 = call-poly <vilib>:"CTRE_Phoenix_MotorController_Get_Enhanced.vi"("PhoenixMotorControlDevRef"=w413) -> ("Percent Output"=w416:dbl)  [unwired: 10 in, 4 out]
        "Voltage" <- w416
        n226 = call-poly <vilib>:"CTRE_Phoenix_MotorController_Get_Enhanced.vi"("PhoenixMotorControlDevRef"=w413, "pidLoopIdx"=u32 0) -> ("Velocity (Raw Sensor Units per 100 ms)"=w412:i32)  [unwired: 10 in, 3 out]
        n227 = Bundle("FWSetpoint"="FWSetpoint", "Velocity (Raw Sensor Units per 100 ms)"=w412) -> (→"Velocity PIDF":T2)  [unwired: 1 in]
        n228 = Bundle("Percent Output"=w416) -> (→"Voltage Output":cluster{"Percent Output":dbl})  [unwired: 1 in]
      }
    }
    n229 = Wait (ms)(milliseconds to wait=u32 10) -> ()  [unwired: 1 out]
  }
  n230 = while {
    stop <- FALSE stop-if-true
    # "Turret PID"
    n231 = global read "MotorsGlobal.vi" "LL Valid Target?"() -> (w431:bool)
    n232 = case shown="True" w431 {
      frame False {
      }
      frame True {
        n233 = global read "MotorsGlobal.vi" "TurretMode"() -> (w434:T27)
        n234 = case shown="\"Automatic\"" w434 {
          frame "Static", Default {
            n235 = global write "MotorsGlobal.vi" "TurretOutput"(0.0 ("FlywheelOutput")) -> ()
          }
          frame "Manual" {
            n236 = global read "JoysticksGlobal.vi" "OpAxe 4"() -> (w437:dbl)
            n237 = call "60Percent.vi"("In"=w437) -> ("Out"=w436:dbl)  [unwired: 9 in]
            n238 = global write "MotorsGlobal.vi" "TurretOutput"(w436) -> ()
          }
          frame "Automatic" {
            n239 = global read "MotorsGlobal.vi" "LimelightX"() -> (w465:dbl)
            n240 = Absolute Value(x=w465) -> (abs(x)=w440:dbl)
            n241 = Greater?(x=w440, y=5.0) -> (0:w463:bool)
            n242 = Greater?(x=w440, y=2.0) -> (0:w458:bool)
            n243 = Subtract(x="TASetpoint", y=w465) -> (x-y=w473:dbl)
            n244 = Less?(x=w440, y=10.0) -> (x < y?=w438:bool)
            "LTAGainsON?" <- w438
            n245 = Absolute Value(x=w473) -> (abs(x)=w472:dbl)
            n246 = Select(t="MTARange", s=w458, f="LTARange") -> (s? t:f=w462:cluster{"output high":dbl, "output low":dbl})
            n247 = Select(t="LTAGains", s=w438, f="TAGains") -> (s? t:f=w441:T3)
            n248 = Select(t="HTARange", s=w463, f=w462) -> (s? t:f=w466:cluster{"output high":dbl, "output low":dbl})
            n249 = Less?(x=w472, y=3.0) -> (x < y?=w470:bool)
            n250 = call "TurretAnglePID.vi"("TAGains"=w441, "TARange"=w466, "TADisable Range"="TADisable Range", "TAIntegral Range"="TAIntegral Range", "TAProcess variable"=w465, "TASetpoint"="TASetpoint") -> ("TAoutput"=w457:dbl)  [unwired: 5 in]
            n251 = Select(t=0.0, s=w470, f="Minimum command") -> (s? t:f=w456:dbl)
            n252 = global read "MotorsGlobal.vi" "TurretEncoder"() -> (w454:dbl)
            n253 = Bundle("TASetpoint"="TASetpoint", "LimelightX"=w465) -> (→"Turret PID":cluster{"TASetpoint":dbl, "LimelightX":dbl})  [unwired: 1 in]
            n254 = global read "MotorsGlobal.vi" "TurretEncoder"() -> (w452:dbl)
            n255 = Add(x=w457, y=w456) -> (x+y=w455:dbl)
            "Turret Out" <- w455
            n256 = Negate(x="MaxAngle") -> (-x=w451:dbl)
            n257 = Negate(x=w455) -> (-x=w448:dbl)
            n258 = Greater?(x=w454, y="MaxAngle") -> (0:w450:bool)
            n259 = Less?(x=w452, y=w451) -> (x < y?=w444:bool)
            n260 = Select(t=-0.1, s=w450, f=w448) -> (s? t:f=w449:dbl)
            n261 = Select(t=0.1, s=w444, f=w449) -> (s? t:f=w447:dbl)
            n262 = global write "MotorsGlobal.vi" "TurretOutput"(w447) -> ()
          }
        }
      }
    }
    n263 = Wait (ms)(milliseconds to wait=u32 10) -> ()  [unwired: 1 out]
  }
  n264 = disable-structure shown="Disabled" {
    frame Disabled {
      n265 = while {
        shift-right: _ -> [_]
        shift-left: _ -> [_]
        stop <- _ stop-if-true
        # "Ball counter"
        n266 = case shown="\"More balls\"" {
          selector: _ -> [_ _]
          frame "Start", Default {
          }
          frame "More balls" {
            (unwired) Ball_counter."Start"
          }
        }
      }
    }
    frame Enabled {
    }
  }
